vi "设置项数据.vi"(0 "通用配置输入":T1={"ModBusRTU反馈"=enum."无反馈", "侦听周期"=0, "跳转反馈"=FALSE, "报文记录数量"=0, "客服端新增模式"=enum."单端模式"}, 12 "枚举":enum16{"INI", "写入", "获取"}(ring)) -> (14 "通用配置输出":T1={"ModBusRTU反馈"=enum."无反馈", "侦听周期"=0, "跳转反馈"=FALSE, "报文记录数量"=0, "客服端新增模式"=enum."单端模式"})   [LabVIEW 2019, in "MainPage.lvlib" / "MainPage.lvclass"]
uses:
  MainPage.lvclass
panel:
  # "实际+10ms间隔时间"
  # "达到上限会顶替旧记录"
  # "实际+10ms间隔时间"
  # "达到上限会顶替旧记录"
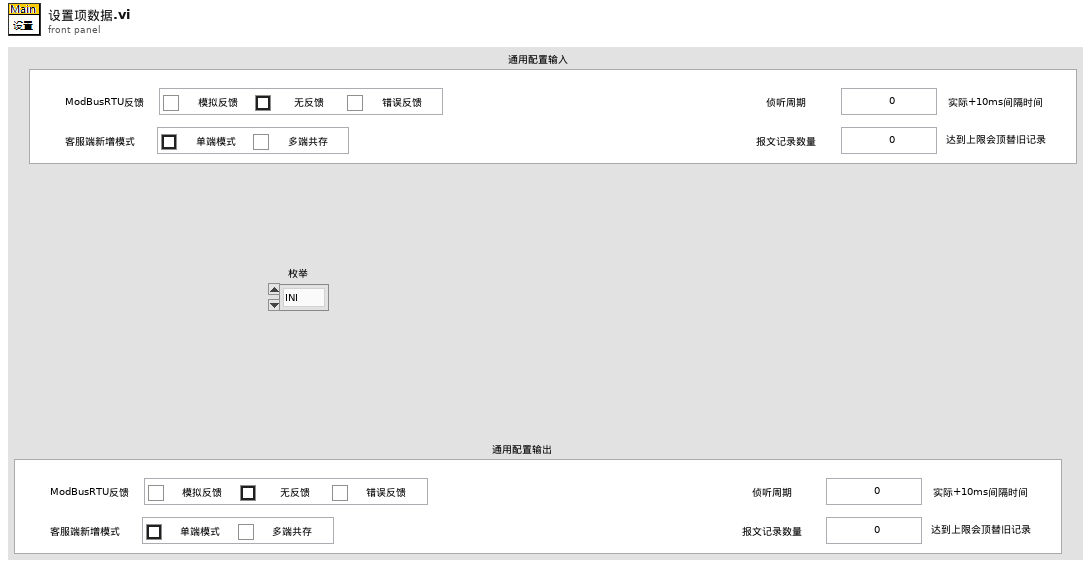
[diagram p1: front panel]
types:
  T1 = typedef "MainPage.lvlib/MainPage.lvclass/通用配置选项.ctl" = cluster{"ModBusRTU反馈":enum32{"模拟反馈", "无反馈", "错误反馈"}, "侦听周期":u32, "跳转反馈":bool, "报文记录数量":u16, "客服端新增模式":enum32{"单端模式", "多端共存"}}
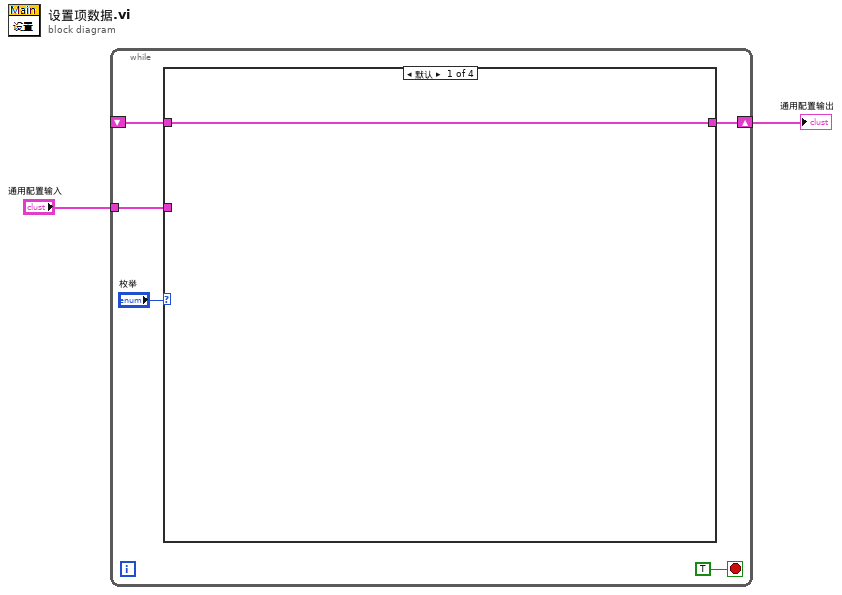
[diagram p0: block diagram]
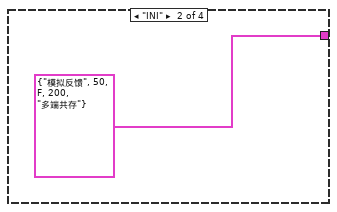
[diagram p2: hidden frame]
diagram:
  n1 = while {
    shift-right: [w4] -> w2
    shift-left: _ -> [w6]
    tunnel: "通用配置输入" -> [w3]
    stop <- TRUE stop-if-true
    n2 = case shown="默认" "枚举" {
      tunnel: w6 -> [w8 _ _ w11]
      tunnel: [w8 T1 {"ModBusRTU反馈"=enum."模拟反馈", "侦听周期"=50, "跳转反馈"=FALSE, "报文记录数量"=200, "客服端新增模式"=enum."多端共存"} ("通用配置输入") w10 w11] -> w4
      tunnel: w3 -> [_ _ w10 _]
      frame Default {
      }
      frame "INI" {
      }
      frame "写入" {
      }
      frame "获取" {
      }
    }
  }
  "通用配置输出" <- w2
